vi "singleTrial_noReturn_HOME.vi"() -> ()   [LabVIEW 2018]
uses:
  <vilib>/Utility/file.llb/Read Delimited Spreadsheet (DBL).vi
  <vilib>/Utility/file.llb/Write Delimited Spreadsheet (I64).vi
panel:
  in  "difficulty":string(combo)="1"
  in  "Maze rotation":string(combo)="clockwise"
  in  "Choice/goal platforms up or down?":string(combo)="up"
  in  "Rat ID":string
  out "choices":i32[][](array[numeric])
  in  "Goal \nplatform":i32
  in  "start platform":i32
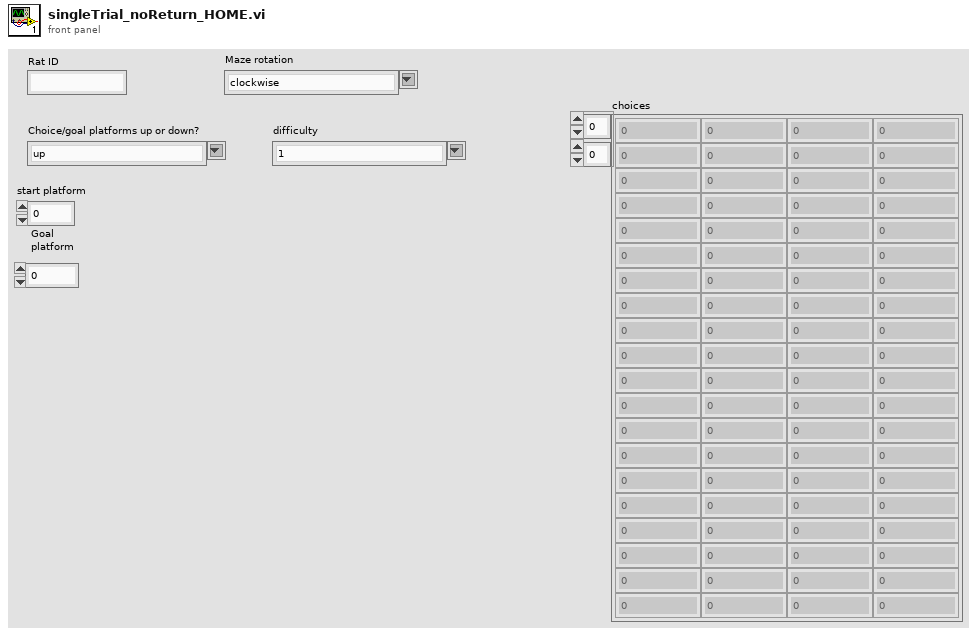
[diagram p1: front panel]
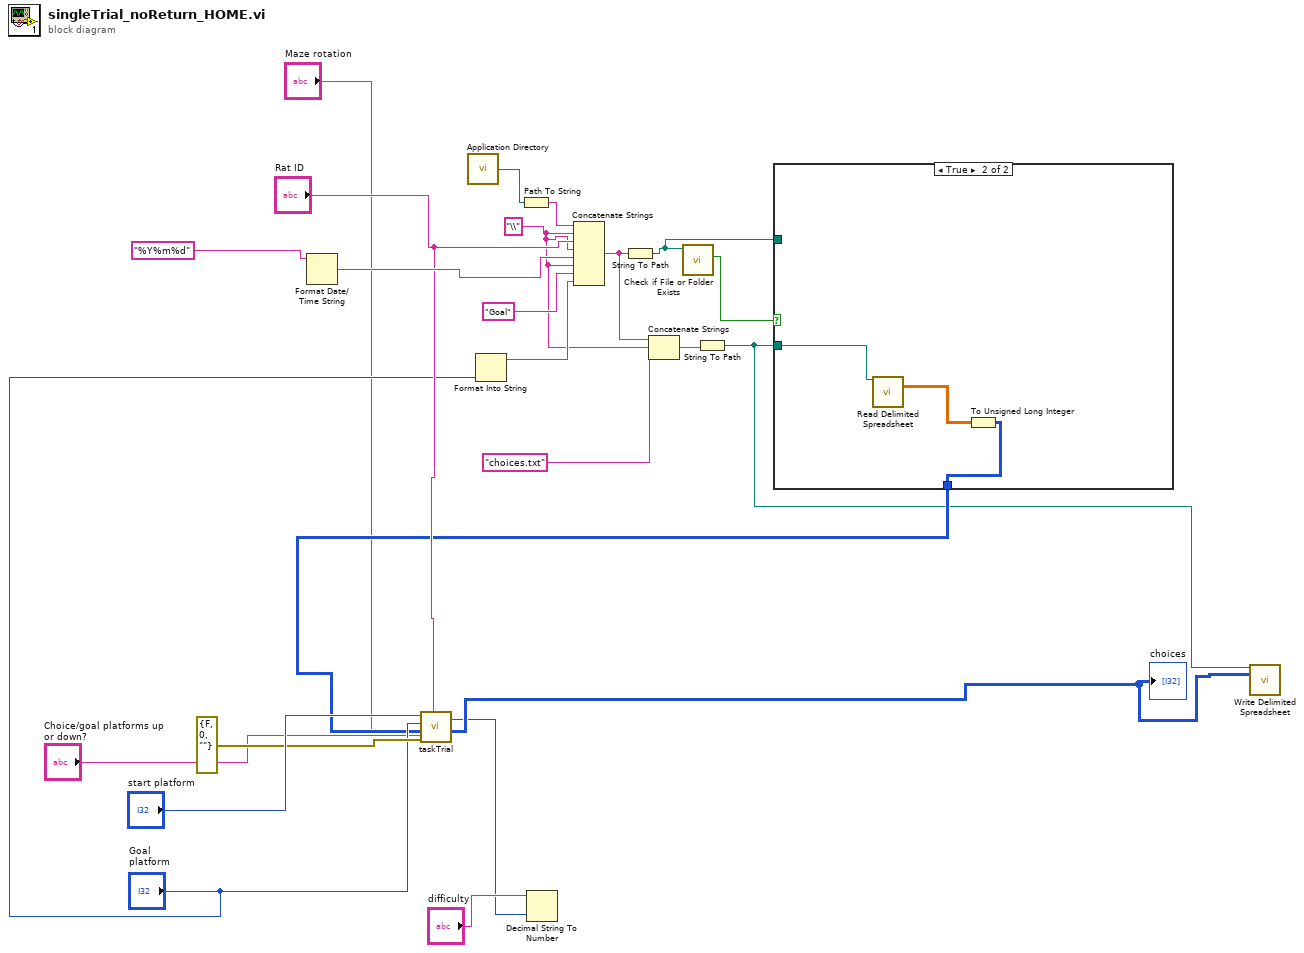
[diagram p0: block diagram]
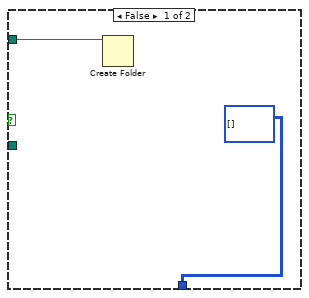
[diagram p2: hidden frame]
diagram:
  w12 = "\\" ("string")
  n1 = Format Date/Time String(time format string (%c)="%Y%m%d" ("time string")) -> (date/time string=w19:string)  [unwired: 2 in]
  n2 = call <vilib>:"Application Directory.vi"() -> ("Application Directory"=w18:path)
  n3 = Format Into String("Goal \nplatform") -> (resulting string=w14:string)  [unwired: 3 in, 1 out]
  n4 = Path To String(path=w18) -> (string=w21:string)
  n5 = Decimal String To Number(string="difficulty") -> (number=w1:i32)  [unwired: 2 in, 1 out]
  n6 = Concatenate Strings(w21, w12, "Rat ID", w12, w19, w12, "Goal" ("string"), w14) -> (w11:string)
  n7 = String To Path(string=w11) -> (path=w7:path)
  n8 = Concatenate Strings(w11, w12, "choices.txt" ("string")) -> (w9:string)
  n9 = call <vilib>:"Check if File or Folder Exists.vi"("path"=w7) -> ("file or folder exists?"=w13:bool)  [unwired: 8 in, 2 out]
  n10 = String To Path(string=w9) -> (path=w6:path)
  n11 = case shown="True" w13 {
    tunnel: w6 -> [_ w28]
    tunnel: [i32[][] [] ("previousChoices") w26] -> w8
    tunnel: w7 -> [w24 _]
    frame False {
      n12 = Create Folder(path (use dialog)=w24) -> ()  [unwired: 2 in, 3 out]
    }
    frame True {
      n13 = call-poly <vilib>:"Read Delimited Spreadsheet.vi"("file path (dialog if empty)"=w28) -> ("all rows"=w27:dbl[][])  [unwired: 9 in, 5 out]
      n14 = To Unsigned Long Integer(number=w27) -> (unsigned 32bit integer=w26:u32[][])
    }
  }
  n15 = call "taskTrial.vi"(4:"Maze rotation", 5:w1, 6:"Choice/goal platforms up or down?", 7:"Rat ID", "error in (no error)"=errorcluster {"status"=FALSE, "code"=0, "source"=""}, "previousChoices"=w8, "Goal \nplatform"="Goal \nplatform", "start platform"="start platform") -> ("previousChoices updated"=w4:i32[][])  [unwired: 1 in, 2 out]
  "choices" <- w4
  n16 = call-poly <vilib>:"Write Delimited Spreadsheet.vi"("file path (dialog if empty)"=w6, "2D data"=w4) -> ()  [unwired: 12 in, 2 out]
